vi "HCC Hawk Viper Data.vi"(8 "Error In":errorcluster, 11 "Diagnostic Data Output":T1) -> (0 "Error Out":errorcluster, 3 "Data W\\Header":string[][](array[string]))   [LabVIEW 2016]
uses:
  Type Definitions/ViperHawk/ViperHawk Diagnostic Data.ctl
  <vilib>/Utility/error.llb/whitespace.ctl
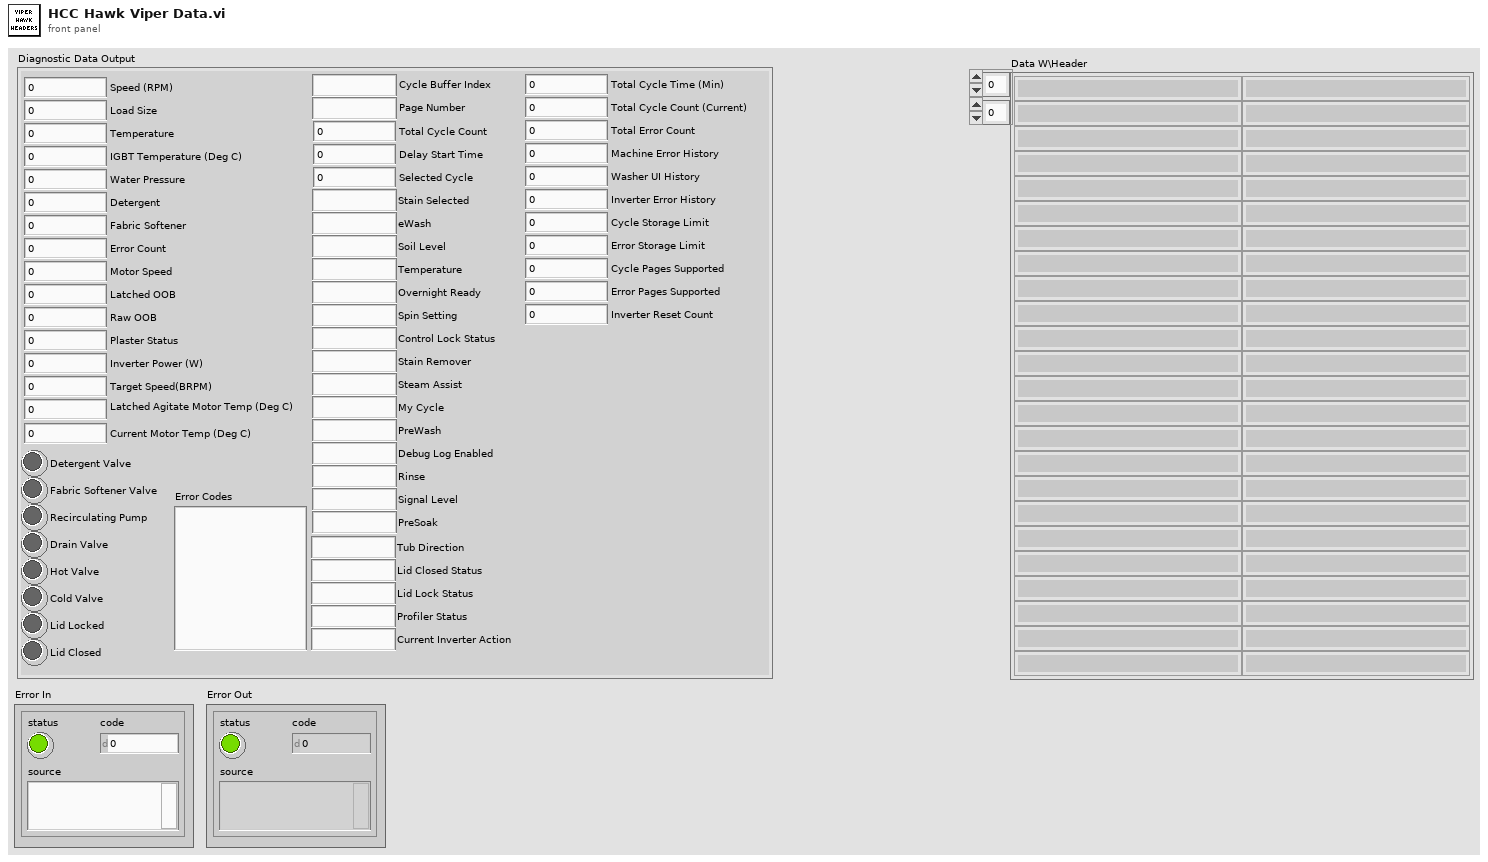
[diagram p1: front panel]
types:
  T1 = typedef "ViperHawk Diagnostic Data.ctl" = cluster{"Speed (RPM)":u32, "Load Size":u32, "Temperature":u32, "Water Pressure":dbl, "Detergent":u32, "Fabric Softener":u32, "Tub Direction":string, "Detergent Valve":bool, "Fabric Softener Valve":bool, "Recirculating Pump":bool, "Drain Valve":bool, "Hot Valve":bool, "Cold Valve":bool, "Lid Closed Status":string, "Lid Lock Status":string, "Error Count":u32, "IGBT Temperature (Deg C)":u32, "Motor Speed":u32, "Latched OOB":u32, "Raw OOB":u32, "Plaster Status":u32, "Inverter Power (W)":u32, "Target Speed(BRPM)":u32, "Latched Agitate Motor Temp (Deg C)":u32, "Current Motor Temp (Deg C)":u32, "Profiler Status":string, "Current Inverter Action":string, "Error Codes":string, "Lid Locked":bool, "Lid Closed":bool, "9E Diagnostic Data":cluster{"Total Cycle Time (Min)":u32, "Total Cycle Count (Current)":u16, "Total Error Count":u16, "Machine Error History":u32, "Washer UI History":u32, "Inverter Error History":u32, "Cycle Storage Limit":u8, "Error Storage Limit":u8, "Cycle Pages Supported":u8, "Error Pages Supported":u8, "Inverter Reset Count":u16}, "9F Diagnostic Data":cluster{"Cycle Buffer Index":string, "Page Number":string, "Total Cycle Count":u32, "Delay Start Time":u32, "Stain Selected":string, "Selected Cycle":u32, "eWash":string, "Soil Level":string, "Temperature":string, "Overnight Ready":string, "Spin Setting":string, "Control Lock Status":string, "Stain Remover":string, "Steam Assist":string, "My Cycle":string, "PreWash":string, "Debug Log Enabled":string, "Rinse":string, "Signal Level":string, "PreSoak":string}}
  T2 = typedef "whitespace.ctl" = u16
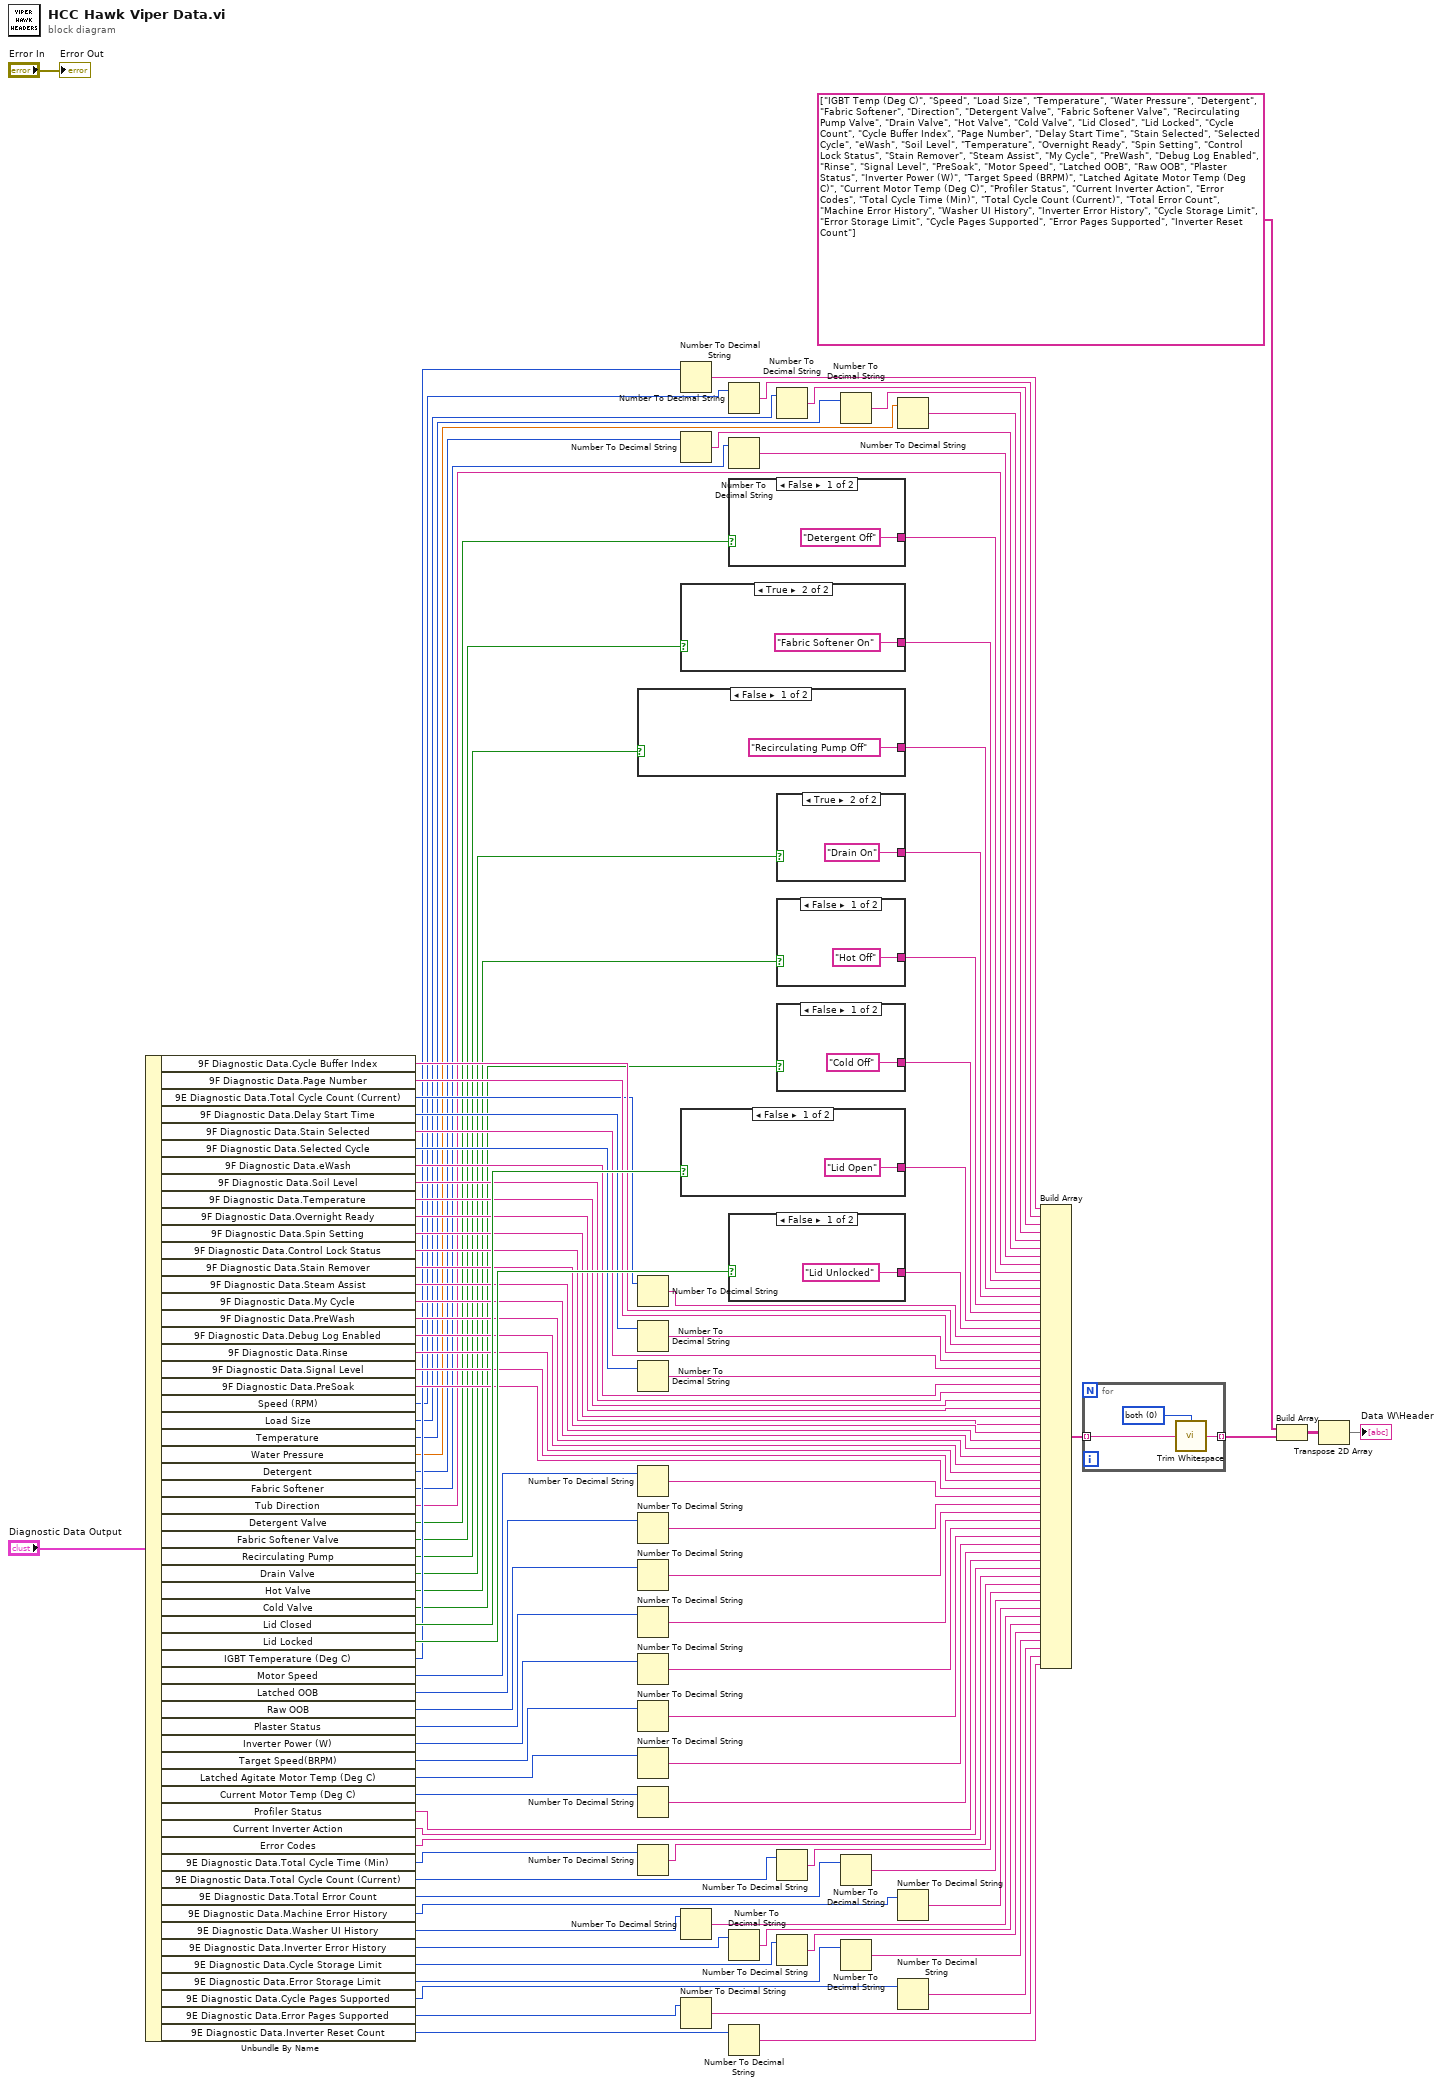
[diagram p0: block diagram]
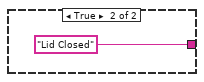
[diagram p2: hidden frame]
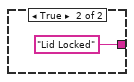
[diagram p3: hidden frame]
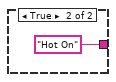
[diagram p4: hidden frame]
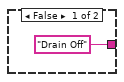
[diagram p5: hidden frame]
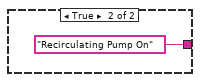
[diagram p6: hidden frame]
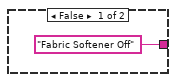
[diagram p7: hidden frame]
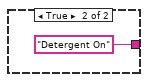
[diagram p8: hidden frame]
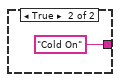
[diagram p9: hidden frame]
diagram:
  n1 = Unbundle By Name("Diagnostic Data Output") -> ("9F Diagnostic Data.Cycle Buffer Index"=w74:string, "9F Diagnostic Data.Page Number"=w75:string, "9E Diagnostic Data.Total Cycle Count (Current)"=w32:u16, "9F Diagnostic Data.Delay Start Time"=w33:u32, "9F Diagnostic Data.Stain Selected"=w36:string, "9F Diagnostic Data.Selected Cycle"=w34:u32, "9F Diagnostic Data.eWash"=w38:string, "9F Diagnostic Data.Soil Level"=w39:string, "9F Diagnostic Data.Temperature"=w40:string, "9F Diagnostic Data.Overnight Ready"=w41:string, "9F Diagnostic Data.Spin Setting"=w42:string, "9F Diagnostic Data.Control Lock Status"=w43:string, "9F Diagnostic Data.Stain Remover"=w44:string, "9F Diagnostic Data.Steam Assist"=w45:string, "9F Diagnostic Data.My Cycle"=w46:string, "9F Diagnostic Data.PreWash"=w47:string, "9F Diagnostic Data.Debug Log Enabled"=w48:string, "9F Diagnostic Data.Rinse"=w49:string, "9F Diagnostic Data.Signal Level"=w50:string, "9F Diagnostic Data.PreSoak"=w52:string, "Speed (RPM)"=w30:u32, "Load Size"=w29:u32, "Temperature"=w28:u32, "Water Pressure"=w27:dbl, "Detergent"=w26:u32, "Fabric Softener"=w25:u32, "Tub Direction"=w24:string, "Detergent Valve"=w18:bool, "Fabric Softener Valve"=w19:bool, "Recirculating Pump"=w20:bool, "Drain Valve"=w21:bool, "Hot Valve"=w22:bool, "Cold Valve"=w23:bool, "Lid Closed"=w101:bool, "Lid Locked"=w102:bool, "IGBT Temperature (Deg C)"=w31:u32, "Motor Speed"=w53:u32, "Latched OOB"=w54:u32, "Raw OOB"=w55:u32, "Plaster Status"=w56:u32, "Inverter Power (W)"=w57:u32, "Target Speed(BRPM)"=w58:u32, "Latched Agitate Motor Temp (Deg C)"=w59:u32, "Current Motor Temp (Deg C)"=w60:u32, "Profiler Status"=w69:string, "Current Inverter Action"=w70:string, "Error Codes"=w71:string, "9E Diagnostic Data.Total Cycle Time (Min)"=w76:u32, "9E Diagnostic Data.Total Cycle Count (Current)"=w77:u16, "9E Diagnostic Data.Total Error Count"=w78:u16, "9E Diagnostic Data.Machine Error History"=w79:u32, "9E Diagnostic Data.Washer UI History"=w80:u32, "9E Diagnostic Data.Inverter Error History"=w81:u32, "9E Diagnostic Data.Cycle Storage Limit"=w82:u8, "9E Diagnostic Data.Error Storage Limit"=w83:u8, "9E Diagnostic Data.Cycle Pages Supported"=w84:u8, "9E Diagnostic Data.Error Pages Supported"=w85:u8, "9E Diagnostic Data.Inverter Reset Count"=w86:u16)
  n2 = case shown="False" w20 {
    tunnel: ["Recirculating Pump Off" "Recirculating Pump On"] -> w11
    frame False {
    }
    frame True {
    }
  }
  n3 = Number To Decimal String(number=w32) -> (decimal integer string=w16:string)  [unwired: 1 in]
  n4 = Number To Decimal String(number=w33) -> (decimal integer string=w35:string)  [unwired: 1 in]
  n5 = Number To Decimal String(number=w34) -> (decimal integer string=w37:string)  [unwired: 1 in]
  n6 = Number To Decimal String(number=w53) -> (decimal integer string=w61:string)  [unwired: 1 in]
  n7 = Number To Decimal String(number=w54) -> (decimal integer string=w62:string)  [unwired: 1 in]
  n8 = Number To Decimal String(number=w55) -> (decimal integer string=w63:string)  [unwired: 1 in]
  n9 = Number To Decimal String(number=w56) -> (decimal integer string=w64:string)  [unwired: 1 in]
  n10 = Number To Decimal String(number=w57) -> (decimal integer string=w65:string)  [unwired: 1 in]
  n11 = Number To Decimal String(number=w58) -> (decimal integer string=w66:string)  [unwired: 1 in]
  n12 = Number To Decimal String(number=w59) -> (decimal integer string=w67:string)  [unwired: 1 in]
  n13 = Number To Decimal String(number=w60) -> (decimal integer string=w68:string)  [unwired: 1 in]
  n14 = Number To Decimal String(number=w76) -> (decimal integer string=w87:string)  [unwired: 1 in]
  n15 = Number To Decimal String(number=w31) -> (decimal integer string=w2:string)  [unwired: 1 in]
  n16 = Number To Decimal String(number=w26) -> (decimal integer string=w7:string)  [unwired: 1 in]
  n17 = case shown="True" w19 {
    tunnel: ["Fabric Softener Off" "Fabric Softener On"] -> w10
    frame False {
    }
    frame True {
    }
  }
  n18 = case shown="False" w101 {
    tunnel: ["Lid Open" "Lid Closed"] -> w99
    frame False {
    }
    frame True {
    }
  }
  n19 = Number To Decimal String(number=w80) -> (decimal integer string=w91:string)  [unwired: 1 in]
  n20 = Number To Decimal String(number=w85) -> (decimal integer string=w96:string)  [unwired: 1 in]
  n21 = Number To Decimal String(number=w30) -> (decimal integer string=w3:string)  [unwired: 1 in]
  n22 = Number To Decimal String(number=w25) -> (decimal integer string=w8:string)  [unwired: 1 in]
  n23 = case shown="False" w18 {
    tunnel: ["Detergent Off" "Detergent On"] -> w9
    frame False {
    }
    frame True {
    }
  }
  n24 = case shown="False" w102 {
    tunnel: ["Lid Unlocked" "Lid Locked"] -> w100
    frame False {
    }
    frame True {
    }
  }
  n25 = Number To Decimal String(number=w81) -> (decimal integer string=w92:string)  [unwired: 1 in]
  n26 = Number To Decimal String(number=w86) -> (decimal integer string=w97:string)  [unwired: 1 in]
  n27 = Number To Decimal String(number=w29) -> (decimal integer string=w4:string)  [unwired: 1 in]
  n28 = case shown="True" w21 {
    tunnel: ["Drain Off" "Drain On"] -> w12
    frame False {
    }
    frame True {
    }
  }
  n29 = case shown="False" w22 {
    tunnel: ["Hot Off" "Hot On"] -> w13
    frame False {
    }
    frame True {
    }
  }
  n30 = case shown="False" w23 {
    tunnel: ["Cold Off" "Cold On"] -> w14
    frame False {
    }
    frame True {
    }
  }
  n31 = Number To Decimal String(number=w77) -> (decimal integer string=w88:string)  [unwired: 1 in]
  n32 = Number To Decimal String(number=w82) -> (decimal integer string=w93:string)  [unwired: 1 in]
  n33 = Number To Decimal String(number=w28) -> (decimal integer string=w5:string)  [unwired: 1 in]
  n34 = Number To Decimal String(number=w78) -> (decimal integer string=w89:string)  [unwired: 1 in]
  n35 = Number To Decimal String(number=w83) -> (decimal integer string=w94:string)  [unwired: 1 in]
  n36 = Number To Decimal String(number=w27) -> (decimal integer string=w6:string)  [unwired: 1 in]
  n37 = Number To Decimal String(number=w79) -> (decimal integer string=w90:string)  [unwired: 1 in]
  n38 = Number To Decimal String(number=w84) -> (decimal integer string=w95:string)  [unwired: 1 in]
  n39 = Build Array(w2, w3, w4, w5, w6, w7, w8, w24, w9, w10, w11, w12, w13, w14, w99, w100, w16, w74, w75, w35, w36, w37, w38, w39, w40, w41, w42, w43, w44, w45, w46, w47, w48, w49, w50, w52, w61, w62, w63, w64, w65, w66, w67, w68, w69, w70, w71, w87, w88, w89, w90, w91, w92, w93, w94, w95, w96, w97) -> (w72:string[])
  n40 = for {
    tunnel: w72 -> [w121] mode=indexing
    tunnel: [w119] -> w73 mode=indexing
    w120 = T2 0 items=["both", "start of string", "end of string"] ("location (both)")
    n41 = call <vilib>:"Trim Whitespace.vi"("string"=w121, "location (both)"=w120) -> ("trimmed string"=w119:string)
  }
  n42 = Build Array(string[] ["IGBT Temp (Deg C)", "Speed", "Load Size", "Temperature", "Water Pressure", "Detergent", "Fabric Softener", "Direction", "Detergent Valve", "Fabric Softener Valve", "Recirculating Pump Valve", "Drain Valve", "Hot Valve", "Cold Valve", "Lid Closed", "Lid Locked", "Cycle Count", "Cycle Buffer Index", "Page Number", "Delay Start Time", "Stain Selected", "Selected Cycle", "eWash", "Soil Level", "Temperature", "Overnight Ready", "Spin Setting", "Control Lock Status", "Stain Remover", "Steam Assist", "My Cycle", "PreWash", "Debug Log Enabled", "Rinse", "Signal Level", "PreSoak", "Motor Speed", "Latched OOB", "Raw OOB", "Plaster Status", "Inverter Power (W)", "Target Speed (BRPM)", "Latched Agitate Motor Temp (Deg C)", "Current Motor Temp (Deg C)", "Profiler Status", "Current Inverter Action", "Error Codes", "Total Cycle Time (Min)", "Total Cycle Count (Current)", "Total Error Count", "Machine Error History", "Washer UI History", "Inverter Error History", "Cycle Storage Limit", "Error Storage Limit", "Cycle Pages Supported", "Error Pages Supported", "Inverter Reset Count"], w73) -> (w15:string[][])
  n43 = Transpose 2D Array(2D array=w15) -> (transposed array=→"Data W\\Header":string[][])
  "Error Out" <- "Error In"
